vi "farenheit_to_celsius.vi"() -> ()   [LabVIEW 2020]
panel:
  in  "farenheit":dbl(slide) scale=-200.0..300.0
  out "Thermometer":dbl(slide) scale=0.0..100.0
  # "c=(f-32)%1.8"
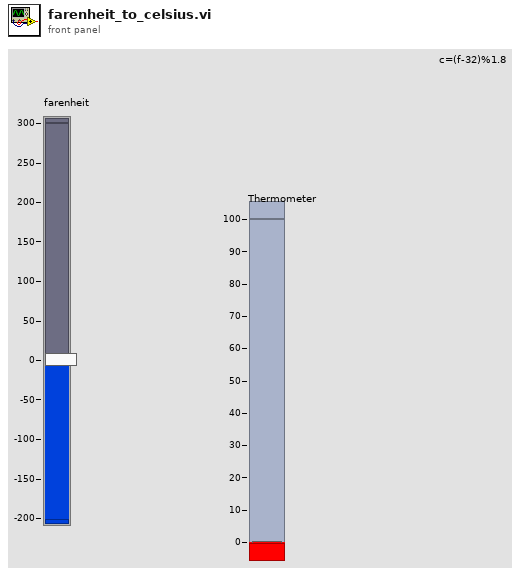
[diagram p1: front panel]
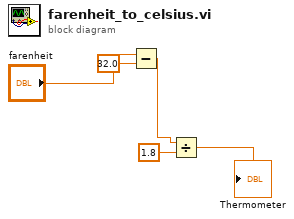
[diagram p0: block diagram]
diagram:
  n1 = Subtract(x="farenheit", y=32.0) -> (x-y=w4:dbl)
  n2 = Divide(x=w4, y=1.8) -> (x/y=→"Thermometer":dbl)
